vi "IR2100_get_rdg.vi"(1 "Address":T1) -> (3 "Comment":string, 5 "Reading":dbl format="%.3f")   [LabVIEW 2010]
uses:
  ADAM Client/Sub VIs/ADAM Controls/Address.ctl
  <vilib>/Instr/serial.llb/serpConfig.vi
panel:
  out "error out":errorcluster
  out "Channel":u16(ring) items=["Current Value", "Mode", "Status", "Gas type", "Unit type", "Version", "Gain", "Disable LED", "Solenoid I/O", "Address", "Ratio", "Baud Rate", "Data Format", "Not Used", "Not Used", "Not Used", "Not Used", "Not Used", "Not Used", "Not Used", "Not Used", "Not Used", "Not Used", "Not Used", "Not Used", "Not Used", "Not Used", "Not Used", "Not Used", "Not Used", "Not Used", "Not Used", "# Rcv Errors", "% Activity Rate", "# Function Err", "# Start Errors", "# Register Err.", "# CRC hi Errors", "# CRC lo Errors", "# Overrun Err.", "# Noise Errors", "# Framing Err", "Not Used", "Not Used", "Not Used", "Clear Errors"]
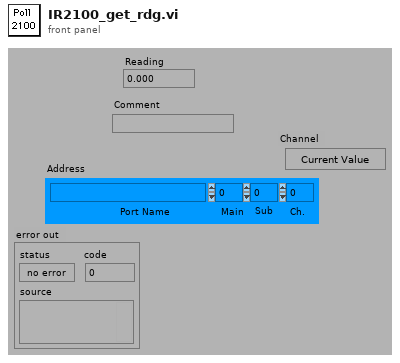
[diagram p1: front panel]
types:
  T1 = typedef "Address.ctl" = cluster{"Main":i32, "Ch.":i32, "Sub":i32, "Port Name":string}
  T2 = enum16{"01 Read digital output status", "02 Read digital input status", "03 Read output registers", "04 Read input registers", "05 Write single digital output", "06 Write single output register", "15 Write multiple digital outputs", "16 Write multiple output registers"}
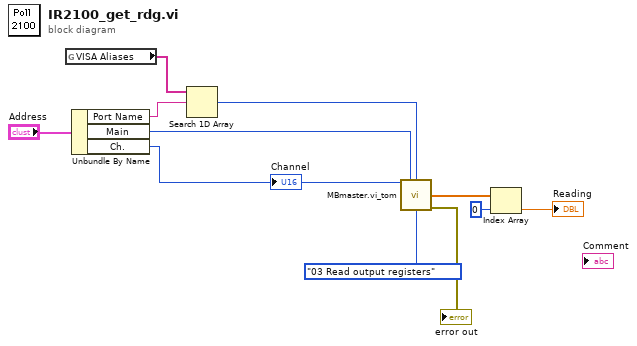
[diagram p0: block diagram]
diagram:
  n1 = global read "serpConfig.vi" "VISA Aliases"() -> (w6:string[])
  n2 = Unbundle By Name("Address") -> ("Port Name"=w5:string, "Main"=w3:i32, "Ch."=w2:i32)
  "Channel" <- w2
  n3 = Search 1D Array(1D array=w6, element=w5) -> (index of element=w4:i32)  [unwired: 1 out]
  n4 = call "MBmaster.vi_tom.vi"("Register address (0)"=w2, "Modbus address (1)"=w3, "port number"=w4, "ModBus Function"=T2."03 Read output registers") -> ("Process values"=w10:dbl[], "error out"=→"error out":errorcluster)  [unwired: 5 in, 5 out]
  n5 = Index Array(array=w10, index=0) -> (element=→"Reading":dbl)
